vi "Packet Encode.vi"(8 "error in (no error)":errorcluster, 11 "Direction in":refnum<class "Direction.lvclass">) -> (0 "error out":errorcluster, 2 "Data":u8[](array[numeric]), 3 "Direction out":refnum<class "Direction.lvclass">)   [LabVIEW 2019, in "Direction.lvclass"]
uses:
  Direction.lvclass
  TCP Packet/Packet.lvclass
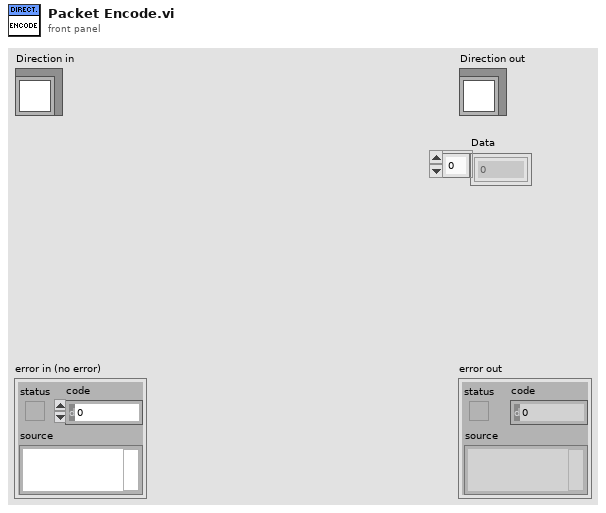
[diagram p1: front panel]
types:
  T1 = typedef "Direction STYP.ctl" = enum16{"Up", "Down", "Left", "Right"}
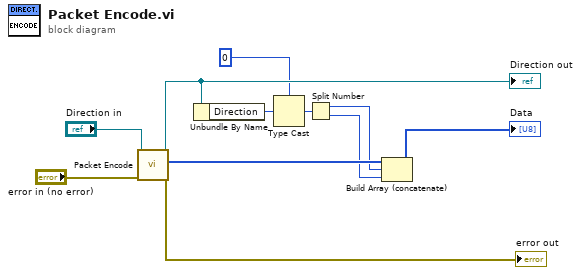
[diagram p0: block diagram]
diagram:
  n1 = call-parent "Packet Encode.vi"("error in (no error)"="error in (no error)", "Packet in"="Direction in") -> ("error out"=→"error out":errorcluster, "Data"=w4:u8[], "Packet out"=w8:refnum<class "Direction.lvclass">)  [unwired: 7 in]
  "Direction out" <- w8
  n2 = Unbundle By Name(w8) -> ("Direction"=w7:T1)
  n3 = Type Cast(type=u16 0, x=w7) -> (*(type *) &x=w5:u16)
  n4 = Split Number(x=w5) -> (hi(x)=w3:u8, lo(x)=w2:u8)
  n5 = Build Array (concatenate)(w4, w3, w2) -> (→"Data":u8[])
